vi "Autonomous Independent.vi"() -> ()   [LabVIEW 2015]
doc: "This VI is called when autonomous begins, and will automatically be terminated when autonomous ends. You can carry out timed or sensor driven robot movement independently without needing to return to the caller."
uses:
  <vilib>/Rock Robotics/WPI/Utilities/WPI_GetSetVariantRefNum.vi
  <vilib>/Rock Robotics/Network Tables/NT Write Numeric Array.vi
  <vilib>/Rock Robotics/Network Tables/NT Read Boolean.vi
  <vilib>/Rock Robotics/WPI/RobotDrive/WPI_RobotDriveArcadeDrive_Standard(NoSaturation).vi
  <vilib>/Rock Robotics/Network Tables/NT Write Boolean.vi
  <vilib>/Rock Robotics/Network Tables/NT Write Number.vi
  <vilib>/Rock Robotics/Network Tables/NT Read Number.vi
panel:
  in  "Ticks to Turn Right":i32
  in  "To goto the edge of the goal":i32=10
  in  "Value to Raise to.":dbl=70.0
  out "POT Sensor Meter 2":dbl(knob) scale=78.0..98.0
  out "POT Sensor Value 2":dbl
  in  "Ticks to Turn Left":i32=8
  in  "Distance to goto the Defence":i32=36
  in  "Ticks to Drive forwad close to the turnning Point":i32=45
  in  "Desides the Distance for Loop 1":i32=16
  out "VAR-Storage-1":dbl
  out "Low Switch":bool
  out "High Switch":bool
  out "POT Sensor Meter":dbl(knob) scale=78.0..98.0
  out "POT Sensor Value":dbl
  # "Also This value is the \nTotal amount of ticks not Turns!\n\nSo 6 Ticks EQU 1 Full Turn."
  # "Remeber to Right Click:\nData Operatoins -> Make Current Value Default"
  # "LOOP 1 - LOOP 1 - LOOP 1 - LOOP 1 - LOOP 1 - LOOP 1 - LOOP 1 - LOOP 1 - LOOP 1 - LOOP 1 - LOOP 1"
  # "DRIVE PAST THE DEFENCE"
  # "LOOP 2  - LOOP 2  - LOOP 2  - LOOP 2  - LOOP 2  - LOOP 2 -  LOOP 2 - LOOP 2  - LOOP 2  - LOOP 2 - LOOP 2"
  # "THIS IS TO DRIVE PAST THE DEFENCE AND TRY TO SHOT"
  # "LOOP 3  - LOOP 3  - LOOP 3  - LOOP 3  - LOOP 3  - LOOP 3  - LOOP 3  - LOOP 3  - LOOP 3  - LOOP 3 - LOOP 3"
  # "THIS LOOP IS FOR DRIVING \nTHE EDGE OF THE DEFFENCE"
  # "Be sure to right-click and choose Data Operations>>Make Current Value default if you want to save the array values with the VI"
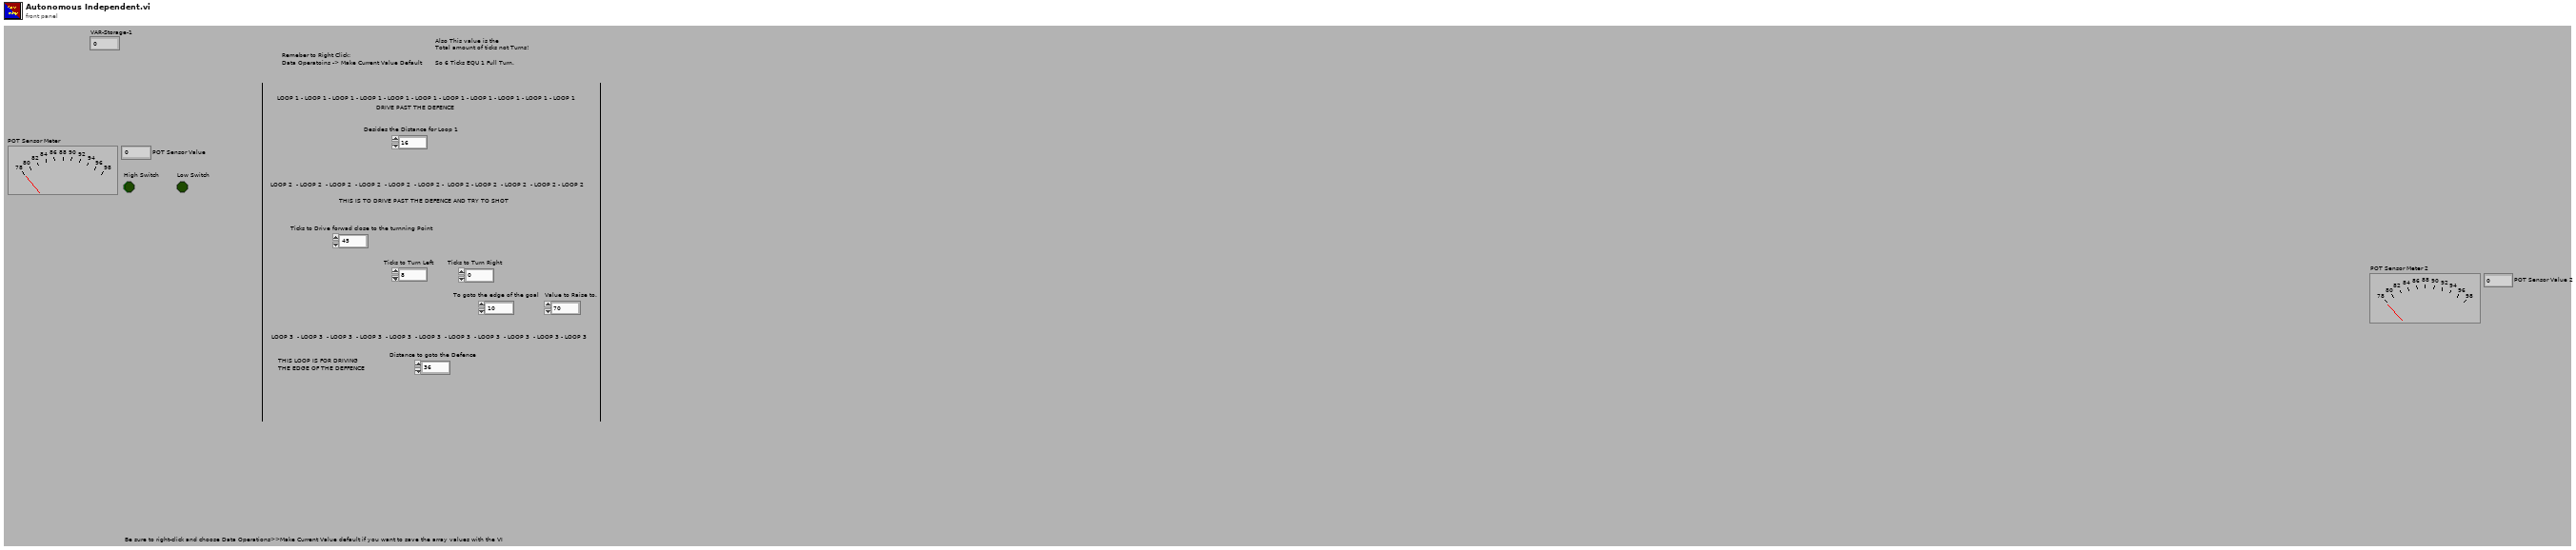
[diagram p1: front panel]
types:
  T1 = typedef "WPI_JoystickDevRef.ctl" = cluster{"Device":T2}
  T2 = typedef "WPI_JoystickDeviceEnum.ctl" = enum16{"USB 0", "USB 1", "USB 2", "USB 3", "USB 4", "USB 5"}
  T3 = typedef "WPI_RobotDriveDevRef.ctl" = cluster{"DevStatus":errorcluster, "Motors[]":T4[], "Square Inputs":bool, "Max Output":dbl}
  T4 = typedef "WPI_MotorControlDeviceRef.ctl" = cluster{"DeviceStatus":errorcluster, "Type":T5, "PWM":cluster{"PWM Channel":T6, "DeadBand":T7}, "CAN":cluster{"Device Number":u8, "Control Mode":T8, "Semaphore":T9, "Max Vout":dbl, "TalonSRX Control Mode":T10}, "Invert":bool}
  T5 = typedef "WPI_MotorControlType.ctl" = enum16{"PWM", "CAN", "CANTalonSRX"}
  T6 = typedef "FPGA_DIOPWMChannel.ctl" = enum8{"PWM 0", "PWM 1", "PWM 2", "PWM 3", "PWM 4", "PWM 5", "PWM 6", "PWM 7", "PWM 8", "PWM 9", "PWM MXP 0", "PWM MXP 1", "PWM MXP 2", "PWM MXP 3", "PWM MXP 4", "PWM MXP 5", "PWM MXP 6", "PWM MXP 7", "PWM MXP 8", "PWM MXP 9", "Invalid"}
  T7 = typedef "WPI_PWMDeadband.ctl" = cluster{"Name":string, "maxPositivePwm":i32, "minPositivePwm":i32, "centerPwm":i32, "maxNegativePwm":i32, "minNegativePwm":i32, "angularRange":u16}
  T8 = typedef "WPI_CANJaguar_ControlMode.ctl" = enum8{"Percent VBus", "Current", "Speed", "Position", "Voltage"}
  T9 = typedef "Semaphore RefNum" = refnum<k1>
  T10 = typedef "WPI_CANTalonSRX_APIControlMode.ctl" = enum8{"Percent VBus", "Speed", "Position", "Slave", "Unchanged / Invalid", "Voltage Compensation", "Current", "Motion Profile"}
  T11 = typedef "WPI_CounterDevRef.ctl" = cluster{"DevStatus":errorcluster, "CntIndex":T12}
  T12 = typedef "FPGA_CounterCtrSystemIndex.ctl" = enum8{"Ctr 0", "Ctr 1", "Ctr 2", "Ctr 3", "Ctr 4", "Ctr 5", "Ctr 6", "Ctr 7", "Invalid"}
  T13 = typedef "WPI_SwitchDevRef.ctl" = cluster{"DevStatus":errorcluster, "DIO Channel":T14, "CntIndex":T12, "Normally Closed":bool}
  T14 = typedef "FPGA_DIOChannel.ctl" = enum8{"DIO 0", "DIO 1", "DIO 2", "DIO 3", "DIO 4", "DIO 5", "DIO 6", "DIO 7", "DIO 8", "DIO 9", "DIO MXP 0", "DIO MXP 1", "DIO MXP 2", "DIO MXP 3", "DIO MXP 4", "DIO MXP 5", "DIO MXP 6", "DIO MXP 7", "DIO MXP 8", "DIO MXP 9", "DIO MXP 10", "DIO MXP 11", "DIO MXP 12", "DIO MXP 13", "DIO MXP 14", "DIO MXP 15", "Invalid"}
  T15 = typedef "WPI_PotentiometerDevRef.ctl" = cluster{"DevStatus":errorcluster, "Analog Channel":T16, "Invert Output":bool}
  T16 = typedef "FPGA_AIChannel.ctl" = enum8{"AI 0", "AI 1", "AI 2", "AI 3", "AI MXP 0", "AI MXP 1", "AI MXP 2", "AI MXP 3", "Invalid"}
  T17 = typedef "WPI_ServoDeviceRef.ctl" = cluster{"DeviceStatus":errorcluster, "PWM Channel":T6, "DeadBand":T7}
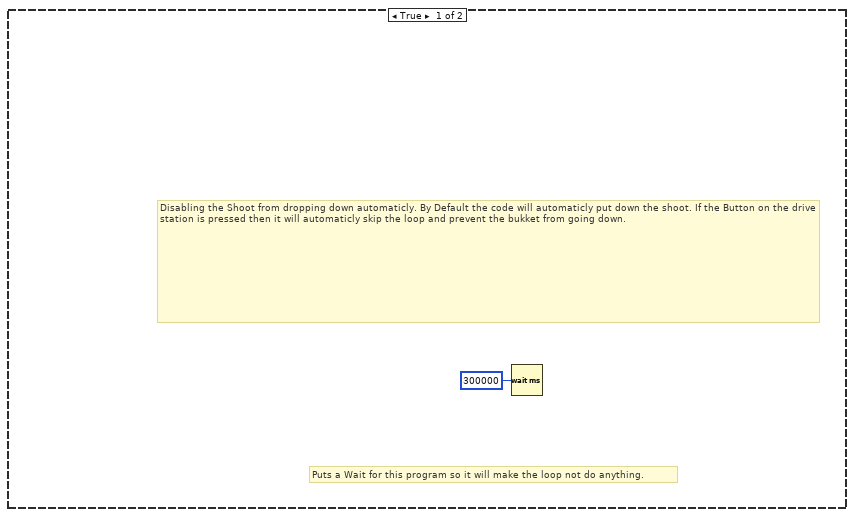
[diagram p2: hidden frame]
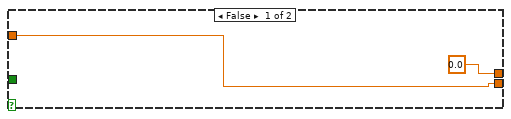
[diagram p3: hidden frame]
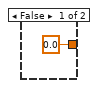
[diagram p4: hidden frame]
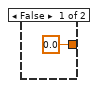
[diagram p6: hidden frame]
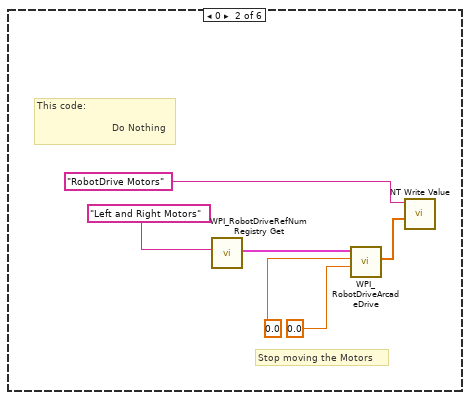
[diagram p9: hidden frame]
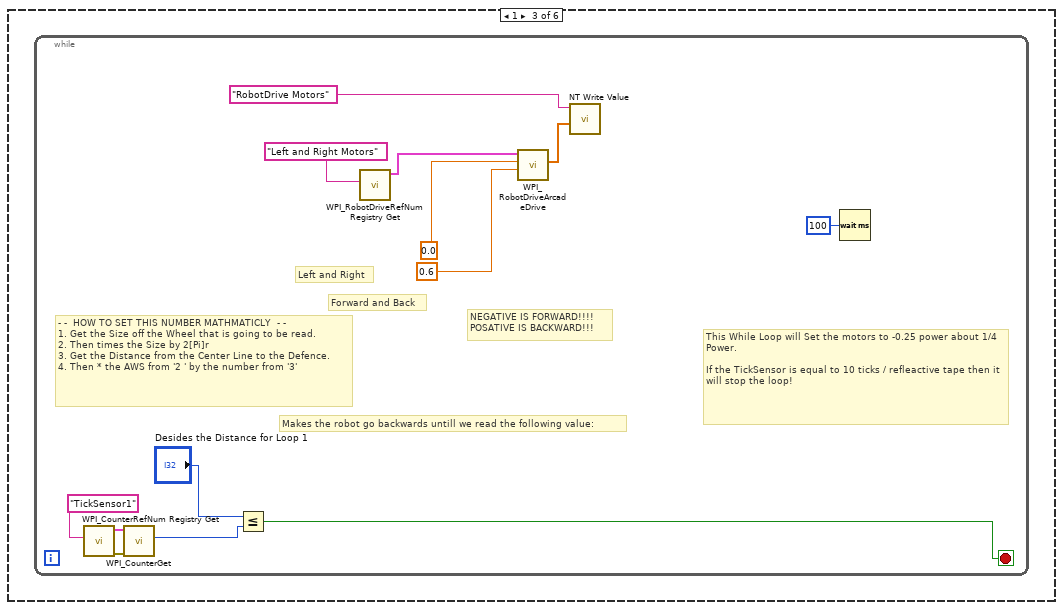
[diagram p10: hidden frame]
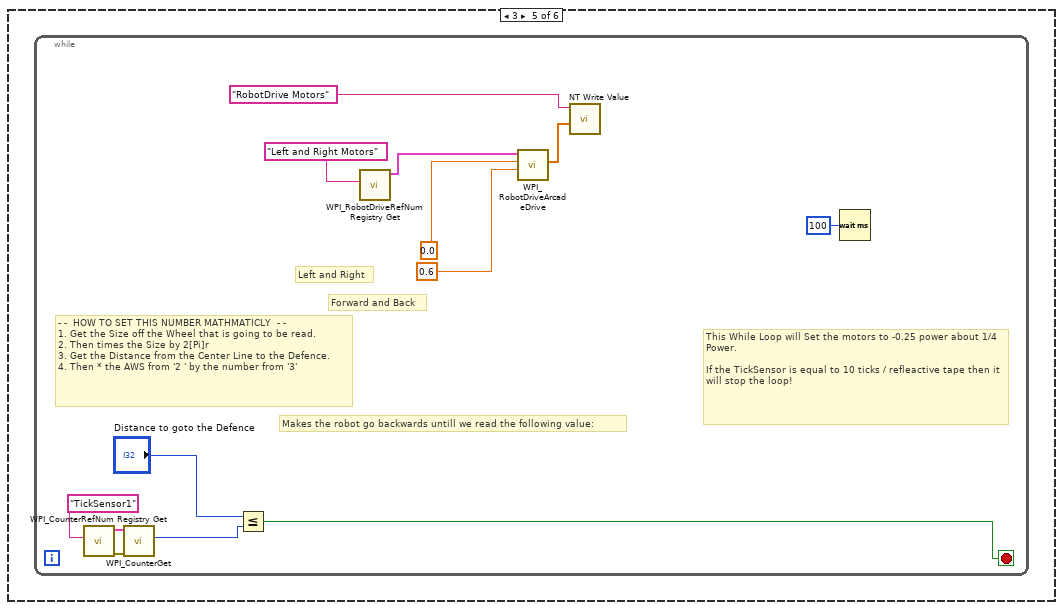
[diagram p11: hidden frame]
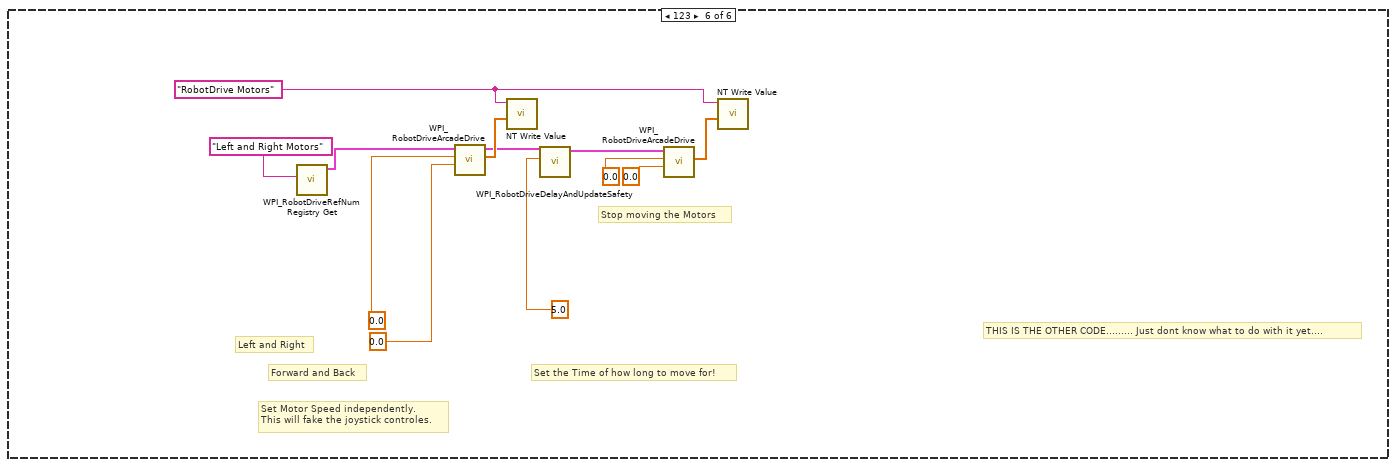
[diagram p12: hidden frame]
diagram:
  (unwired) "This function is run in parallel when the autonomous period begins. It will be terminated automatically when the period ends.\n\nNote that all Driver Station inputs are automatically latched and will not change once auto begins."
  # "Every 20ms, report that we are running autonomous\ncode. Loop will abort the same time as the VI."
  # "This gives you the joystick value\nthat is often the throttle"
  # "This tells you the driver position\nand alliance color"
  n1 = while {
    stop <- FALSE stop-if-true
    n2 = call <vilib>:"WPI_DriverStationReport Robot Code State.vi"("Autonomous"=TRUE) -> ()  [unwired: 10 in, 1 out]
    n3 = Wait (ms)(milliseconds to wait=u32 20) -> ()  [unwired: 1 out]
  }
  n4 = call <vilib>:"WPI_DriverStationGet Alliance Info.vi"() -> ()  [unwired: 12 out]
  n5 = call <vilib>:"WPI_JoystickRefNum Registry Get.vi"("refnum name"="Joystick 0") -> ("JoystickDevRef"=w5:T1)  [unwired: 1 in, 9 out]
  n6 = call-poly <vilib>:"NT Read Value.vi"("Name"="Auto Selector") -> ()  [unwired: 9 in, 2 out]
  n7 = call <vilib>:"WPI_JoystickGetValues.vi"("JoystickDevRef"=w5) -> ("Axes"=w3:dbl[])  [unwired: 6 in, 4 out]
  n8 = call-poly <vilib>:"NT Write Value.vi"("Numeric Array"=w3, "Name"="Joystick 0/Axes") -> ()  [unwired: 9 in, 1 out]
  n9 = Index Array(array=w3, index=2) -> ()  [unwired: 1 out]
  n10 = flat-sequence {
    frame #0 {
      n11 = call <vilib>:"WPI_RobotDriveRefNum Registry Get.vi"("refnum name"="Left and Right Motors") -> ("RobotDriveDevRef"=w20:T3)  [unwired: 1 in, 9 out]
      n12 = call <vilib>:"WPI_MotorControlRefNum Registry Get.vi"("refnum name"="BPMs") -> ("error out"=w12:errorcluster, "MotorControlDevRef"=w11:T4)  [unwired: 9 in]
      n13 = call <vilib>:"WPI_CounterRefNum Registry Get.vi"("refnum name"="TickSensor2") -> ("error out"=w27:errorcluster, "CounterDevRef"=w26:T11)  [unwired: 9 in]
      n14 = call <vilib>:"WPI_CounterRefNum Registry Get.vi"("refnum name"="TickSensor1") -> ("error out"=w30:errorcluster, "CounterDevRef"=w29:T11)  [unwired: 9 in]
      n15 = call <vilib>:"WPI_CounterRefNum Registry Get.vi"("refnum name"="TickSensor2") -> ("error out"=w18:errorcluster, "CounterDevRef"=w19:T11)  [unwired: 9 in]
      n16 = call <vilib>:"WPI_CounterRefNum Registry Get.vi"("refnum name"="TickSensor1") -> ("error out"=w15:errorcluster, "CounterDevRef"=w16:T11)  [unwired: 9 in]
      n17 = call <vilib>:"WPI_MotorControlSetOutput.vi"("error in (no error)"=w12, "Output"=0.0, "MotorControlDevRef"=w11) -> ()  [unwired: 6 in, 3 out]
      n18 = call <vilib>:"WPI_CounterReset.vi"("error in (no error)"=w27, "CounterDevRef in"=w26) -> ()  [unwired: 8 in, 2 out]
      n19 = call <vilib>:"WPI_CounterReset.vi"("error in (no error)"=w30, "CounterDevRef in"=w29) -> ()  [unwired: 8 in, 2 out]
      n20 = call <vilib>:"WPI_CounterReset.vi"("error in (no error)"=w18, "CounterDevRef in"=w19) -> ()  [unwired: 8 in, 2 out]
      n21 = call <vilib>:"WPI_CounterReset.vi"("error in (no error)"=w15, "CounterDevRef in"=w16) -> ()  [unwired: 8 in, 2 out]
      n22 = call-poly <vilib>:"WPI_RobotDriveArcadeDrive.vi"("Y axis value"=0.0 ("X axis value"), "X axis value"=0.0, "RobotDriveDevRef"=w20) -> ("Motor Values"=w22:dbl[])  [unwired: 1 in, 7 out]
      n23 = call-poly <vilib>:"NT Write Value.vi"("Numeric Array"=w22, "Name"="RobotDrive Motors") -> ()  [unwired: 9 in, 1 out]
    }
    frame #1 {
      n24 = call-poly <vilib>:"NT Read Value.vi"("Default Value"=FALSE, "Name"="DisableLowerOnStart") -> ()  [unwired: 8 in, 2 out]
      n25 = case shown="False" FALSE {
        frame True {
          # "Puts a Wait for this program so it will make the loop not do anything."
          # "Disabling the Shoot from dropping down automaticly. By Default the code will automaticly put down the shoot. If the Button on the drive station is pressed then it will automaticly skip the loop and prevent the bukket from going down."
          n26 = Wait (ms)(milliseconds to wait=u32 300000) -> ()  [unwired: 1 out]
        }
        frame False {
          n27 = while {
            stop <- w37 stop-if-true
            n28 = call <vilib>:"WPI_SwitchRefNum Registry Get.vi"("refnum name"="LowSwitch") -> ("error out"=w60:errorcluster, "SwitchDevRef"=w61:T13)  [unwired: 9 in]
            n29 = call <vilib>:"WPI_SwitchRefNum Registry Get.vi"("refnum name"="HighSwitch") -> ("error out"=w57:errorcluster, "SwitchDevRef"=w58:T13)  [unwired: 9 in]
            n30 = call <vilib>:"WPI_SwitchGetLimitValue.vi"("error in (no error)"=w60, "SwitchDevRef"=w61) -> ("Switch Pressed"=w45:bool)  [unwired: 7 in, 2 out]
            "Low Switch" <- w45
            n31 = call <vilib>:"WPI_SwitchGetLimitValue.vi"("error in (no error)"=w57, "SwitchDevRef"=w58) -> ("Switch Pressed"=w44:bool)  [unwired: 7 in, 2 out]
            "High Switch" <- w44
            n32 = call-poly <vilib>:"NT Write Value.vi"("Boolean"=w45, "Name"="Low Sensor") -> ()  [unwired: 9 in, 1 out]
            n33 = call-poly <vilib>:"NT Write Value.vi"("Boolean"=w44, "Name"="High Sensor") -> ()  [unwired: 9 in, 1 out]
            n34 = Or(x=w45, y=w44) -> (x .or. y?=w62:bool)
            n35 = case shown="True" w62 {
              tunnel: w45 -> [_ w67]
              tunnel: w44 -> [_ w69]
              tunnel: -0.5 ("Axes[1]") -> [w63 w68]
              tunnel: [0.0 ("Axes[1]") w66] -> w51
              tunnel: [w63 w65] -> w50
              frame False {
              }
              frame True {
                n36 = case shown="True" w67 {
                  tunnel: w68 -> [_ w79]
                  tunnel: [0.0 ("Axes[1]") w78] -> w66
                  frame False {
                  }
                  frame True {
                    n37 = Greater?(x=w79, y=0.0) -> (0:w80:bool)
                    n38 = case shown="False" w80 {
                      tunnel: [0.0 ("Axes[1]") w83] -> w78
                      tunnel: w79 -> [_ w83]
                      frame False {
                        # "NO VALUE SENT"
                      }
                      frame True {
                      }
                    }
                  }
                }
                n39 = case shown="True" w69 {
                  tunnel: w68 -> [_ w71]
                  tunnel: [0.0 ("Axes[1]") w72] -> w65
                  frame False {
                  }
                  frame True {
                    n40 = Less?(x=w71, y=0.0) -> (x < y?=w73:bool)
                    n41 = case shown="False" w73 {
                      tunnel: [0.0 ("Axes[1]") w76] -> w72
                      tunnel: w71 -> [_ w76]
                      frame False {
                        # "NO VALUE SENT"
                      }
                      frame True {
                      }
                    }
                  }
                }
              }
            }
            n42 = call <vilib>:"WPI_PotentiometerRefNum Registry Get.vi"("refnum name"="POT Sensor") -> ("error out"=w49:errorcluster, "PotDevRef"=w48:T15)  [unwired: 9 in]
            n43 = call <vilib>:"WPI_PotentiometerGetNormalized.vi"("error in"=w49, "PotDevRef"=w48) -> ("Normalized Value"=w41:dbl)  [unwired: 7 in, 2 out]
            n44 = Multiply(x=w41, y=100.0) -> (x*y=w39:dbl)
            "POT Sensor Value" <- w39
            "POT Sensor Meter" <- w39
            n45 = call-poly <vilib>:"NT Write Value.vi"("Numeric"=w39, "Name"="POT Sensor") -> ()  [unwired: 9 in, 1 out]
            n46 = Add(x=w51, y=w50) -> (x+y=w52:dbl)
            n47 = call <vilib>:"WPI_MotorControlRefNum Registry Get.vi"("refnum name"="Pickup Motor") -> ("error out"=w55:errorcluster, "MotorControlDevRef"=w54:T4)  [unwired: 9 in]
            n48 = local read "Low Switch"() -> (w37:bool)
            n49 = call <vilib>:"WPI_MotorControlSetOutput.vi"("error in (no error)"=w55, "Output"=w52, "MotorControlDevRef"=w54) -> ()  [unwired: 6 in, 3 out]
            n50 = Wait (ms)(milliseconds to wait=u32 100) -> ()  [unwired: 1 out]
          }
        }
      }
    }
    frame #2 {
      # "This tells you the autonomous selected\nfrom the dashboard"
      n51 = call-poly <vilib>:"NT Read Value.vi"("Name"="AutoModeSelector") -> ("Numeric"=w85:dbl)  [unwired: 9 in, 1 out]
      n52 = Wait (ms)(milliseconds to wait=u32 20) -> ()  [unwired: 1 out]
      n53 = case shown="2" w85 {
        frame Default {
          # "You can put your main auto here, or you can right-click on the case and make any\nother frame be the default case."
          # "This is the frame that will execute if no selection is made, or if it is not recognized"
        }
        frame 0 {
          # "Stop moving the Motors"
          # "This code:\n                   \n                         Do Nothing"
          n54 = call <vilib>:"WPI_RobotDriveRefNum Registry Get.vi"("refnum name"="Left and Right Motors") -> ("RobotDriveDevRef"=w87:T3)  [unwired: 1 in, 9 out]
          n55 = call-poly <vilib>:"WPI_RobotDriveArcadeDrive.vi"("Y axis value"=0.0 ("X axis value"), "X axis value"=0.0, "RobotDriveDevRef"=w87) -> ("Motor Values"=w91:dbl[])  [unwired: 1 in, 7 out]
          n56 = call-poly <vilib>:"NT Write Value.vi"("Numeric Array"=w91, "Name"="RobotDrive Motors") -> ()  [unwired: 9 in, 1 out]
        }
        frame 1 {
          n57 = while {
            stop <- w102 stop-if-true
            # "NEGATIVE IS FORWARD!!!!\nPOSATIVE IS BACKWARD!!!"
            # "- -  HOW TO SET THIS NUMBER MATHMATICLY  - - \n1. Get the Size off the Wheel that is going to be read.\n2. Then times the Size by 2[Pi]r\n3. Get the Distance from the Center Line to the Defence.\n4. Then * the AWS from '2 ' by the number from '3'"
            # "Makes the robot go backwards untill we read the following value:"
            # "This While Loop will Set the motors to -0.25 power about 1/4 Power.\n\nIf the TickSensor is equal to 10 ticks / refleactive tape then it will stop the loop!"
            # "Forward and Back"
            # "Left and Right"
            n58 = call <vilib>:"WPI_CounterRefNum Registry Get.vi"("refnum name"="TickSensor1") -> ("error out"=w104:errorcluster, "CounterDevRef"=w103:T11)  [unwired: 9 in]
            n59 = call <vilib>:"WPI_CounterGet.vi"("error in (no error)"=w104, "CounterDevRef in"=w103) -> ("Value"=w94:i32)  [unwired: 4 in, 5 out]
            n60 = Less Or Equal?(x="Desides the Distance for Loop 1", y=w94) -> (x <= y?=w102:bool)
            n61 = call <vilib>:"WPI_RobotDriveRefNum Registry Get.vi"("refnum name"="Left and Right Motors") -> ("RobotDriveDevRef"=w101:T3)  [unwired: 1 in, 9 out]
            n62 = call-poly <vilib>:"WPI_RobotDriveArcadeDrive.vi"("Y axis value"=0.6 ("X axis value"), "X axis value"=0.0, "RobotDriveDevRef"=w101) -> ("Motor Values"=w99:dbl[])  [unwired: 1 in, 7 out]
            n63 = call-poly <vilib>:"NT Write Value.vi"("Numeric Array"=w99, "Name"="RobotDrive Motors") -> ()  [unwired: 9 in, 1 out]
            n64 = Wait (ms)(milliseconds to wait=u32 100) -> ()  [unwired: 1 out]
          }
        }
        frame 2 {
          n65 = flat-sequence {
            frame #0 {
              n66 = while {
                stop <- w121 stop-if-true
                # "- -  HOW TO SET THIS NUMBER MATHMATICLY  - - \n1. Get the Size off the Wheel that is going to be read.\n2. Then times the Size by 2[Pi]r\n3. Get the Distance from the Center Line to the Defence.\n4. Then * the AWS from '2 ' by the number from '3'"
                # "Makes the robot go backwards untill we read the following value:"
                # "This While Loop will Set the motors to -0.25 power about 1/4 Power.\n\nIf the TickSensor is equal to 10 ticks / refleactive tape then it will stop the loop!"
                # "Forward and Back"
                # "Left and Right"
                n67 = call <vilib>:"WPI_CounterRefNum Registry Get.vi"("refnum name"="TickSensor1") -> ("error out"=w123:errorcluster, "CounterDevRef"=w122:T11)  [unwired: 9 in]
                n68 = Wait (ms)(milliseconds to wait=u32 100) -> ()  [unwired: 1 out]
                n69 = call <vilib>:"WPI_CounterGet.vi"("error in (no error)"=w123, "CounterDevRef in"=w122) -> ("Value"=w113:i32)  [unwired: 4 in, 5 out]
                n70 = Less Or Equal?(x="Ticks to Drive forwad close to the turnning Point", y=w113) -> (x <= y?=w121:bool)
                n71 = call <vilib>:"WPI_RobotDriveRefNum Registry Get.vi"("refnum name"="Left and Right Motors") -> ("RobotDriveDevRef"=w120:T3)  [unwired: 1 in, 9 out]
                n72 = call-poly <vilib>:"WPI_RobotDriveArcadeDrive.vi"("Y axis value"=0.6 ("X axis value"), "X axis value"=0.0, "RobotDriveDevRef"=w120) -> ("Motor Values"=w118:dbl[])  [unwired: 1 in, 7 out]
                n73 = call-poly <vilib>:"NT Write Value.vi"("Numeric Array"=w118, "Name"="RobotDrive Motors") -> ()  [unwired: 9 in, 1 out]
              }
              n74 = call <vilib>:"WPI_RobotDriveRefNum Registry Get.vi"("refnum name"="Left and Right Motors") -> ("RobotDriveDevRef"=w106:T3)  [unwired: 1 in, 9 out]
              n75 = call-poly <vilib>:"WPI_RobotDriveArcadeDrive.vi"("Y axis value"=0.0 ("X axis value"), "X axis value"=0.0, "RobotDriveDevRef"=w106) -> ("Motor Values"=w108:dbl[])  [unwired: 1 in, 7 out]
              n76 = call-poly <vilib>:"NT Write Value.vi"("Numeric Array"=w108, "Name"="RobotDrive Motors") -> ()  [unwired: 9 in, 1 out]
            }
            frame #1 {
              n77 = call <vilib>:"WPI_CounterRefNum Registry Get.vi"("refnum name"="TickSensor2") -> ("error out"=w126:errorcluster, "CounterDevRef"=w125:T11)  [unwired: 9 in]
              n78 = call <vilib>:"WPI_CounterRefNum Registry Get.vi"("refnum name"="TickSensor1") -> ("error out"=w129:errorcluster, "CounterDevRef"=w128:T11)  [unwired: 9 in]
              n79 = call <vilib>:"WPI_CounterReset.vi"("error in (no error)"=w126, "CounterDevRef in"=w125) -> ()  [unwired: 8 in, 2 out]
              n80 = call <vilib>:"WPI_CounterReset.vi"("error in (no error)"=w129, "CounterDevRef in"=w128) -> ()  [unwired: 8 in, 2 out]
            }
            frame #2 {
              n81 = while {
                tunnel: [w132] -> _
                stop <- w132 stop-if-true
                # "Forward and Back"
                # "Left and Right"
                n82 = call <vilib>:"WPI_CounterRefNum Registry Get.vi"("refnum name"="TickSensor1") -> ("error out"=w142:errorcluster, "CounterDevRef"=w141:T11)  [unwired: 9 in]
                n83 = call <vilib>:"WPI_CounterGet.vi"("error in (no error)"=w142, "CounterDevRef in"=w141) -> ("Value"=w135:i32)  [unwired: 4 in, 5 out]
                n84 = call <vilib>:"WPI_RobotDriveRefNum Registry Get.vi"("refnum name"="Left and Right Motors") -> ("RobotDriveDevRef"=w140:T3)  [unwired: 1 in, 9 out]
                n85 = Less Or Equal?(x="Ticks to Turn Left", y=w135) -> (x <= y?=w132:bool)
                n86 = call-poly <vilib>:"WPI_RobotDriveArcadeDrive.vi"("Y axis value"=0.0 ("X axis value"), "X axis value"=-0.5, "RobotDriveDevRef"=w140) -> ("Motor Values"=w139:dbl[])  [unwired: 1 in, 7 out]
                n87 = call-poly <vilib>:"NT Write Value.vi"("Numeric Array"=w139, "Name"="RobotDrive Motors") -> ()  [unwired: 9 in, 1 out]
              }
              n88 = Wait (ms)(milliseconds to wait=u32 100) -> ()  [unwired: 1 out]
            }
            frame #3 {
              n89 = call <vilib>:"WPI_RobotDriveRefNum Registry Get.vi"("refnum name"="Left and Right Motors") -> ("RobotDriveDevRef"=w144:T3)  [unwired: 1 in, 9 out]
              n90 = call-poly <vilib>:"WPI_RobotDriveArcadeDrive.vi"("Y axis value"=0.0 ("X axis value"), "X axis value"=0.0, "RobotDriveDevRef"=w144) -> ("Motor Values"=w146:dbl[])  [unwired: 1 in, 7 out]
              n91 = call-poly <vilib>:"NT Write Value.vi"("Numeric Array"=w146, "Name"="RobotDrive Motors") -> ()  [unwired: 9 in, 1 out]
            }
            frame #4 {
              n92 = while {
                tunnel: [w151] -> _
                stop <- w151 stop-if-true
                # "Forward and Back"
                # "Left and Right"
                n93 = call <vilib>:"WPI_CounterRefNum Registry Get.vi"("refnum name"="TickSensor2") -> ("error out"=w161:errorcluster, "CounterDevRef"=w160:T11)  [unwired: 9 in]
                n94 = call <vilib>:"WPI_CounterGet.vi"("error in (no error)"=w161, "CounterDevRef in"=w160) -> ("Value"=w154:i32)  [unwired: 4 in, 5 out]
                n95 = call <vilib>:"WPI_RobotDriveRefNum Registry Get.vi"("refnum name"="Left and Right Motors") -> ("RobotDriveDevRef"=w159:T3)  [unwired: 1 in, 9 out]
                n96 = Less Or Equal?(x="Ticks to Turn Right", y=w154) -> (x <= y?=w151:bool)
                n97 = call-poly <vilib>:"WPI_RobotDriveArcadeDrive.vi"("Y axis value"=0.0 ("X axis value"), "X axis value"=0.5, "RobotDriveDevRef"=w159) -> ("Motor Values"=w158:dbl[])  [unwired: 1 in, 7 out]
                n98 = call-poly <vilib>:"NT Write Value.vi"("Numeric Array"=w158, "Name"="RobotDrive Motors") -> ()  [unwired: 9 in, 1 out]
              }
              n99 = Wait (ms)(milliseconds to wait=u32 100) -> ()  [unwired: 1 out]
            }
            frame #5 {
              n100 = call <vilib>:"WPI_CounterRefNum Registry Get.vi"("refnum name"="TickSensor2") -> ("error out"=w170:errorcluster, "CounterDevRef"=w169:T11)  [unwired: 9 in]
              n101 = call <vilib>:"WPI_CounterRefNum Registry Get.vi"("refnum name"="TickSensor1") -> ("error out"=w173:errorcluster, "CounterDevRef"=w172:T11)  [unwired: 9 in]
              n102 = call <vilib>:"WPI_RobotDriveRefNum Registry Get.vi"("refnum name"="Left and Right Motors") -> ("RobotDriveDevRef"=w168:T3)  [unwired: 1 in, 9 out]
              n103 = call-poly <vilib>:"WPI_RobotDriveArcadeDrive.vi"("Y axis value"=0.0 ("X axis value"), "X axis value"=0.0, "RobotDriveDevRef"=w168) -> ("Motor Values"=w166:dbl[])  [unwired: 1 in, 7 out]
              n104 = call <vilib>:"WPI_CounterReset.vi"("error in (no error)"=w170, "CounterDevRef in"=w169) -> ()  [unwired: 8 in, 2 out]
              n105 = call <vilib>:"WPI_CounterReset.vi"("error in (no error)"=w173, "CounterDevRef in"=w172) -> ()  [unwired: 8 in, 2 out]
              n106 = call-poly <vilib>:"NT Write Value.vi"("Numeric Array"=w166, "Name"="RobotDrive Motors") -> ()  [unwired: 9 in, 1 out]
            }
            frame #6 {
              n107 = while {
                stop <- w184 stop-if-true
                # "- -  HOW TO SET THIS NUMBER MATHMATICLY  - - \n1. Get the Size off the Wheel that is going to be read.\n2. Then times the Size by 2[Pi]r\n3. Get the Distance from the Center Line to the Defence.\n4. Then * the AWS from '2 ' by the number from '3'"
                # "Makes the robot go backwards untill we read the following value:"
                # "This While Loop will Set the motors to -0.25 power about 1/4 Power.\n\nIf the TickSensor is equal to 10 ticks / refleactive tape then it will stop the loop!"
                # "Forward and Back"
                # "Left and Right"
                n108 = call <vilib>:"WPI_CounterRefNum Registry Get.vi"("refnum name"="TickSensor1") -> ("error out"=w186:errorcluster, "CounterDevRef"=w185:T11)  [unwired: 9 in]
                n109 = Wait (ms)(milliseconds to wait=u32 100) -> ()  [unwired: 1 out]
                n110 = call <vilib>:"WPI_CounterGet.vi"("error in (no error)"=w186, "CounterDevRef in"=w185) -> ("Value"=w176:i32)  [unwired: 4 in, 5 out]
                n111 = Less Or Equal?(x="To goto the edge of the goal", y=w176) -> (x <= y?=w184:bool)
                n112 = call <vilib>:"WPI_RobotDriveRefNum Registry Get.vi"("refnum name"="Left and Right Motors") -> ("RobotDriveDevRef"=w183:T3)  [unwired: 1 in, 9 out]
                n113 = call-poly <vilib>:"WPI_RobotDriveArcadeDrive.vi"("Y axis value"=-0.6 ("X axis value"), "X axis value"=0.0, "RobotDriveDevRef"=w183) -> ("Motor Values"=w181:dbl[])  [unwired: 1 in, 7 out]
                n114 = call-poly <vilib>:"NT Write Value.vi"("Numeric Array"=w181, "Name"="RobotDrive Motors") -> ()  [unwired: 9 in, 1 out]
              }
            }
            frame #7 {
              n115 = call <vilib>:"WPI_CounterRefNum Registry Get.vi"("refnum name"="TickSensor2") -> ("error out"=w195:errorcluster, "CounterDevRef"=w194:T11)  [unwired: 9 in]
              n116 = call <vilib>:"WPI_CounterRefNum Registry Get.vi"("refnum name"="TickSensor1") -> ("error out"=w198:errorcluster, "CounterDevRef"=w197:T11)  [unwired: 9 in]
              n117 = call <vilib>:"WPI_CounterReset.vi"("error in (no error)"=w195, "CounterDevRef in"=w194) -> ()  [unwired: 8 in, 2 out]
              n118 = call <vilib>:"WPI_CounterReset.vi"("error in (no error)"=w198, "CounterDevRef in"=w197) -> ()  [unwired: 8 in, 2 out]
              n119 = call <vilib>:"WPI_RobotDriveRefNum Registry Get.vi"("refnum name"="Left and Right Motors") -> ("RobotDriveDevRef"=w193:T3)  [unwired: 1 in, 9 out]
              n120 = call-poly <vilib>:"WPI_RobotDriveArcadeDrive.vi"("Y axis value"=0.0 ("X axis value"), "X axis value"=0.0, "RobotDriveDevRef"=w193) -> ("Motor Values"=w191:dbl[])  [unwired: 1 in, 7 out]
              n121 = call-poly <vilib>:"NT Write Value.vi"("Numeric Array"=w191, "Name"="RobotDrive Motors") -> ()  [unwired: 9 in, 1 out]
            }
            frame #8 {
              n122 = while {
                stop <- w207 stop-if-true
                # "This value will set the pickup motors to lift them up."
                # "This value will be the P.O.T. value. This will stop the Loop from running."
                n123 = call <vilib>:"WPI_PotentiometerRefNum Registry Get.vi"("refnum name"="POT Sensor") -> ("error out"=w213:errorcluster, "PotDevRef"=w212:T15)  [unwired: 9 in]
                n124 = call <vilib>:"WPI_PotentiometerGetNormalized.vi"("error in"=w213, "PotDevRef"=w212) -> ("Normalized Value"=w209:dbl)  [unwired: 7 in, 2 out]
                n125 = Multiply(x=w209, y=100.0) -> (x*y=w206:dbl)
                "POT Sensor Value 2" <- w206
                "POT Sensor Meter 2" <- w206
                n126 = Greater Or Equal?(x=w206, y="Value to Raise to.") -> (x >= y?=w207:bool)
                n127 = call <vilib>:"WPI_MotorControlRefNum Registry Get.vi"("refnum name"="Pickup Motor") -> ("error out"=w205:errorcluster, "MotorControlDevRef"=w204:T4)  [unwired: 9 in]
                n128 = call <vilib>:"WPI_MotorControlSetOutput.vi"("error in (no error)"=w205, "Output"=0.5, "MotorControlDevRef"=w204) -> ()  [unwired: 6 in, 3 out]
                n129 = call-poly <vilib>:"NT Write Value.vi"("Numeric"=w206, "Name"="POT Sensor") -> ()  [unwired: 9 in, 1 out]
                n130 = Wait (ms)(milliseconds to wait=u32 100) -> ()  [unwired: 1 out]
              }
            }
            frame #9 {
              n131 = call <vilib>:"WPI_MotorControlRefNum Registry Get.vi"("refnum name"="BPMs") -> ("error out"=w216:errorcluster, "MotorControlDevRef"=w215:T4)  [unwired: 9 in]
              n132 = call <vilib>:"WPI_MotorControlSetOutput.vi"("error in (no error)"=w216, "Output"=-0.75, "MotorControlDevRef"=w215) -> ()  [unwired: 6 in, 3 out]
            }
            frame #10 {
              n133 = while {
                stop <- w218 stop-if-true
                n134 = call "Elapsed Time"() -> ("Time has Elapsed"=w218:bool)  [unwired: 12 in, 7 out]
              }
            }
            frame #11 {
              # "Sets the Servo to TRUE so it goes to the full open position."
              # "The Low Value"
              n135 = Select(t=0.0, s=TRUE, f=0.3) -> (s? t:f=w220:dbl)
              n136 = call <vilib>:"WPI_ServoRefNum Registry Get.vi"("refnum name"="Servo 1") -> ("error out"=w224:errorcluster, "ServoDeviceRef"=w223:T17)  [unwired: 9 in]
              n137 = call <vilib>:"WPI_ServoSetPosition.vi"("error in (no error)"=w224, "Position"=w220, "ServoDeviceRef"=w223) -> ()  [unwired: 7 in, 2 out]
            }
          }
        }
        frame 3 {
          n138 = while {
            stop <- w235 stop-if-true
            # "- -  HOW TO SET THIS NUMBER MATHMATICLY  - - \n1. Get the Size off the Wheel that is going to be read.\n2. Then times the Size by 2[Pi]r\n3. Get the Distance from the Center Line to the Defence.\n4. Then * the AWS from '2 ' by the number from '3'"
            # "Makes the robot go backwards untill we read the following value:"
            # "This While Loop will Set the motors to -0.25 power about 1/4 Power.\n\nIf the TickSensor is equal to 10 ticks / refleactive tape then it will stop the loop!"
            # "Forward and Back"
            # "Left and Right"
            n139 = call <vilib>:"WPI_CounterRefNum Registry Get.vi"("refnum name"="TickSensor1") -> ("error out"=w237:errorcluster, "CounterDevRef"=w236:T11)  [unwired: 9 in]
            n140 = call <vilib>:"WPI_CounterGet.vi"("error in (no error)"=w237, "CounterDevRef in"=w236) -> ("Value"=w227:i32)  [unwired: 4 in, 5 out]
            n141 = Less Or Equal?(x="Distance to goto the Defence", y=w227) -> (x <= y?=w235:bool)
            n142 = call <vilib>:"WPI_RobotDriveRefNum Registry Get.vi"("refnum name"="Left and Right Motors") -> ("RobotDriveDevRef"=w234:T3)  [unwired: 1 in, 9 out]
            n143 = call-poly <vilib>:"WPI_RobotDriveArcadeDrive.vi"("Y axis value"=0.6 ("X axis value"), "X axis value"=0.0, "RobotDriveDevRef"=w234) -> ("Motor Values"=w232:dbl[])  [unwired: 1 in, 7 out]
            n144 = call-poly <vilib>:"NT Write Value.vi"("Numeric Array"=w232, "Name"="RobotDrive Motors") -> ()  [unwired: 9 in, 1 out]
            n145 = Wait (ms)(milliseconds to wait=u32 100) -> ()  [unwired: 1 out]
          }
        }
        frame 123 {
          w249 = "RobotDrive Motors" ("Name")
          # "THIS IS THE OTHER CODE......... Just dont know what to do with it yet...."
          # "Forward and Back"
          # "Left and Right"
          # "Set Motor Speed independently.\nThis will fake the joystick controles."
          # "Set the Time of how long to move for!"
          # "Stop moving the Motors"
          n146 = call <vilib>:"WPI_RobotDriveRefNum Registry Get.vi"("refnum name"="Left and Right Motors") -> ("RobotDriveDevRef"=w250:T3)  [unwired: 1 in, 9 out]
          n147 = call-poly <vilib>:"WPI_RobotDriveArcadeDrive.vi"("Y axis value"=0.0 ("X axis value"), "X axis value"=0.0, "RobotDriveDevRef"=w250) -> ("Motor Values"=w248:dbl[], "RobotDriveDevRef"=w242:T3)  [unwired: 1 in, 6 out]
          n148 = call-poly <vilib>:"NT Write Value.vi"("Numeric Array"=w248, "Name"=w249) -> ()  [unwired: 9 in, 1 out]
          n149 = call <vilib>:"WPI_RobotDriveDelayAndUpdateSafety.vi"("Delay (s)"=5.0, "RobotDriveDevRef"=w242) -> ("RobotDriveDevRef 2"=w241:T3)  [unwired: 8 in, 1 out]
          n150 = call-poly <vilib>:"WPI_RobotDriveArcadeDrive.vi"("Y axis value"=0.0 ("X axis value"), "X axis value"=0.0, "RobotDriveDevRef"=w241) -> ("Motor Values"=w247:dbl[])  [unwired: 1 in, 7 out]
          n151 = call-poly <vilib>:"NT Write Value.vi"("Numeric Array"=w247, "Name"=w249) -> ()  [unwired: 9 in, 1 out]
        }
      }
    }
    frame #3 {
      n152 = call <vilib>:"WPI_RobotDriveRefNum Registry Get.vi"("refnum name"="Left and Right Motors") -> ("RobotDriveDevRef"=w261:T3)  [unwired: 1 in, 9 out]
      n153 = call <vilib>:"WPI_MotorControlRefNum Registry Get.vi"("refnum name"="BPMs") -> ("error out"=w253:errorcluster, "MotorControlDevRef"=w252:T4)  [unwired: 9 in]
      n154 = call <vilib>:"WPI_CounterRefNum Registry Get.vi"("refnum name"="TickSensor2") -> ("error out"=w259:errorcluster, "CounterDevRef"=w260:T11)  [unwired: 9 in]
      n155 = call <vilib>:"WPI_CounterRefNum Registry Get.vi"("refnum name"="TickSensor1") -> ("error out"=w256:errorcluster, "CounterDevRef"=w257:T11)  [unwired: 9 in]
      n156 = call <vilib>:"WPI_MotorControlSetOutput.vi"("error in (no error)"=w253, "Output"=0.0, "MotorControlDevRef"=w252) -> ()  [unwired: 6 in, 3 out]
      n157 = call <vilib>:"WPI_CounterReset.vi"("error in (no error)"=w259, "CounterDevRef in"=w260) -> ()  [unwired: 8 in, 2 out]
      n158 = call <vilib>:"WPI_CounterReset.vi"("error in (no error)"=w256, "CounterDevRef in"=w257) -> ()  [unwired: 8 in, 2 out]
      n159 = call-poly <vilib>:"WPI_RobotDriveArcadeDrive.vi"("Y axis value"=0.0 ("X axis value"), "X axis value"=0.0, "RobotDriveDevRef"=w261) -> ("Motor Values"=w263:dbl[])  [unwired: 1 in, 7 out]
      n160 = call-poly <vilib>:"NT Write Value.vi"("Numeric Array"=w263, "Name"="RobotDrive Motors") -> ()  [unwired: 9 in, 1 out]
    }
  }
